vi "Parte3_Medicion Remota.vi"() -> ()   [LabVIEW 2020]
uses:
  <vilib>/httpClient/LabVIEWHTTPClient.lvlib
panel:
  out "Temperatura":dbl
  out "Luz lateral":bool
  out "Luz frontal":bool
  out "Fecha":string
  in  "stop":bool
  out "body GET":string
  out "headers GET":string
  out "error out":errorcluster
  out "Humedad":dbl
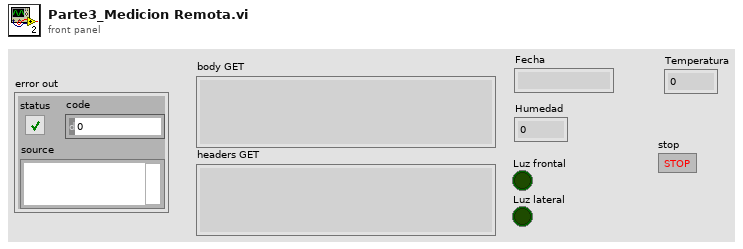
[diagram p1: front panel]
types:
  T1 = cluster{"Humedad":dbl, "Fecha":string, "Luz frontal":bool, "Luz lateral":bool, "Temperatura":dbl}
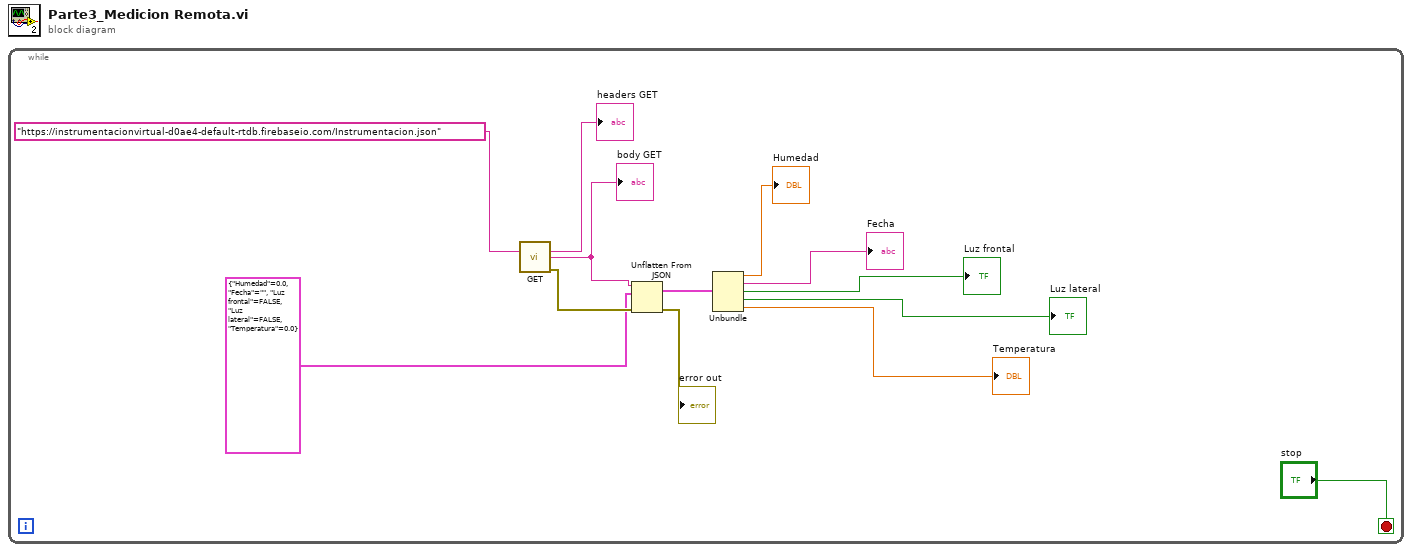
[diagram p0: block diagram]
diagram:
  n1 = while {
    stop <- "stop" stop-if-true
    n2 = call <vilib>:"GET.vi"("url"="https://instrumentacionvirtual-d0ae4-default-rtdb.firebaseio.com/Instrumentacion.json") -> ("headers"=→"headers GET":string, "body"=w10:string, "error out"=w9:errorcluster)  [unwired: 11 in, 1 out]
    "body GET" <- w10
    n3 = Unflatten From JSON(JSON string=w10, type and defaults=T1 {"Humedad"=0.0, "Fecha"="", "Luz frontal"=FALSE, "Luz lateral"=FALSE, "Temperatura"=0.0}, error in (no error)=w9) -> (value=w6:T1, error out=→"error out":errorcluster)  [unwired: 4 in]
    n4 = Unbundle "Unbundle"(w6) -> ("Humedad"=→"Humedad":dbl, "Fecha"=→"Fecha":string, "Luz frontal"=→"Luz frontal":bool, "Luz lateral"=→"Luz lateral":bool, "Temperatura"=→"Temperatura":dbl)
  }
